vi "DecodificaAO.vi"(4 "ForzaAO_PLC":refnum<vi>, 6 "ForzaAO_Cdaq":refnum<vi>, 7 "Caratteristiche Caricate":string[][](array[string]), 8 "AO non scalati IN":T5, 9 "AO PLCs in":T4, 10 "statoAO_Cdaq in":T9, 11 "Cluster SET AO":T6) -> (0 "AO PLCs out":T4, 1 "exit":bool, 3 "statoAO_Cdaq out":T9, 5 "AO non scalati OUT":T5)   [LabVIEW 2019]
uses:
  controls/StatoAO_cdaq.ctl
  SET ARRAY AO.ctl
  SET SINGLE AO.ctl
  AO List.ctl
  TypeDef/Lista AO sistema.ctl
  controls/statoAO_plc_1.ctl
  controls/statoAO_plc_2.ctl
  controls/statoAO_plc_3.ctl
  GlobalForzaUscite.vi
  Global dati targa SINUSPENTA.vi
  Global config keb.vi
  GlobalAOInterfaccia.vi
panel:
  out "Numeric":i32
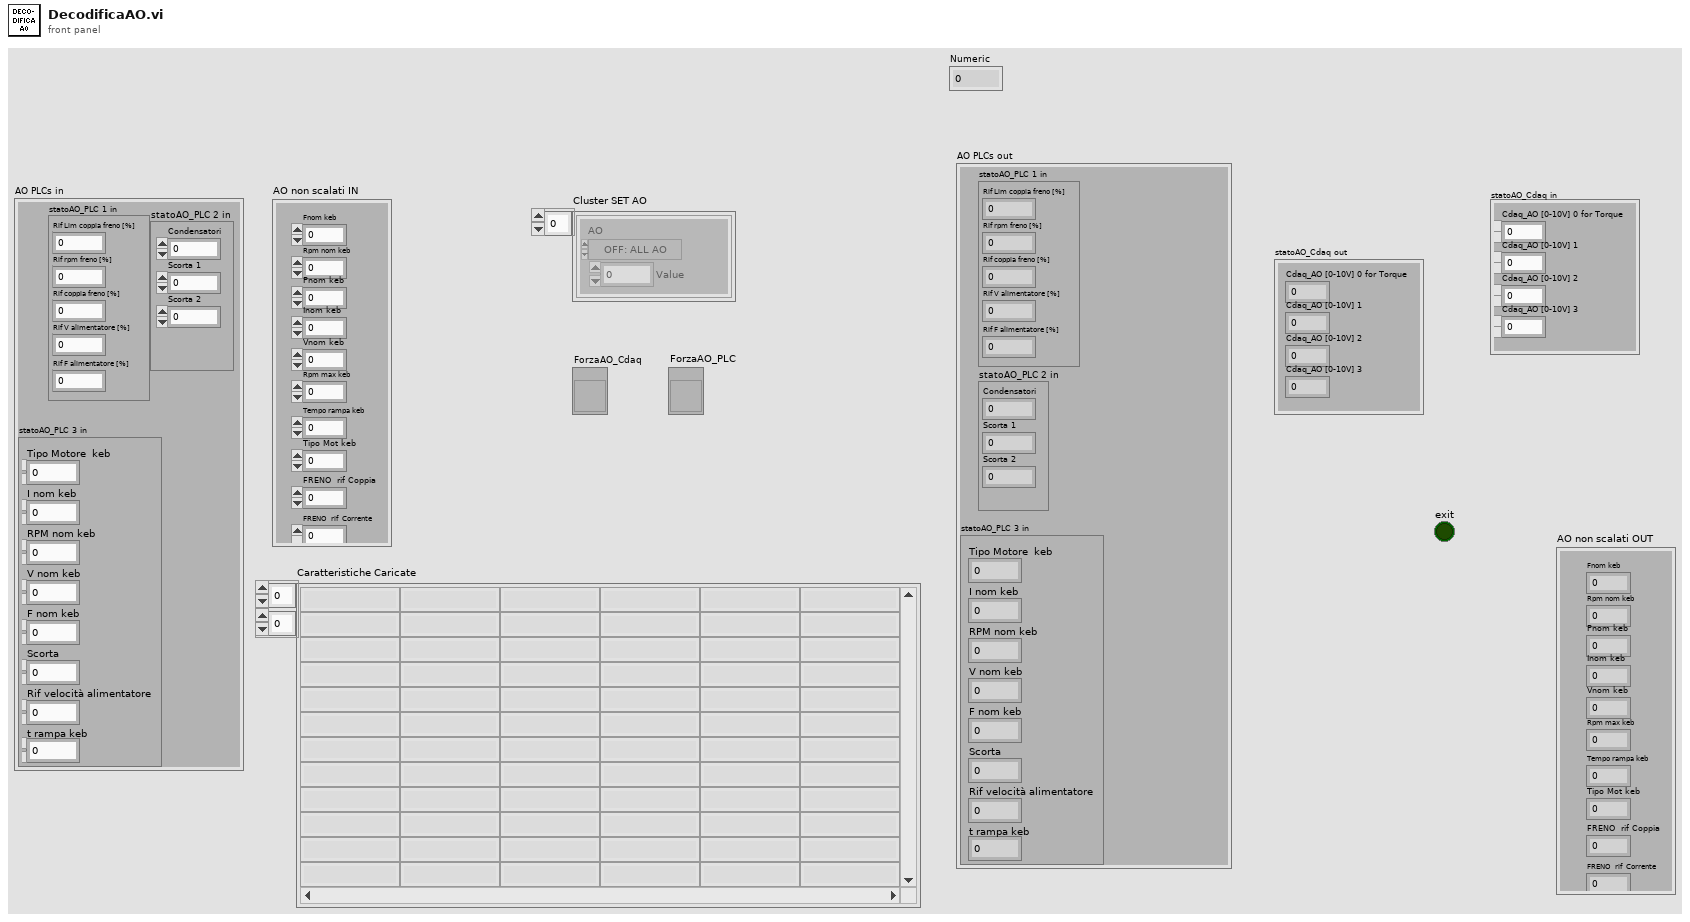
[diagram p1: front panel]
types:
  T1 = typedef "statoAO_plc_1.ctl" = cluster{"Rif Lim coppia freno [%]":dbl, "Rif rpm freno [%]":dbl, "Rif coppia freno [%]":dbl, "Rif V alimentatore [%]":dbl, "Rif F alimentatore [%]":dbl}
  T2 = typedef "statoAO_plc_2.ctl" = cluster{"Condensatori":dbl, "Scorta 1":dbl, "Scorta 2":dbl}
  T3 = typedef "statoAO_plc_3.ctl" = cluster{"Rif velocità alimentatore":dbl, "Scorta":dbl, "Tipo Motore  keb":dbl, "I nom keb":dbl, "RPM nom keb":dbl, "V nom keb":dbl, "F nom keb":dbl, "t rampa keb":dbl}
  T4 = cluster{"statoAO_PLC 1 in":T1, "statoAO_PLC 2 in":T2, "statoAO_PLC 3 in":T3}
  T5 = typedef "Lista AO sistema.ctl" = cluster{"FRENO1 rif vel":dbl, "FRENO1 rif Coppia":dbl, "FRENO2 rif vel":dbl, "FRENO2 rif Coppia":dbl, "ALIM1 rif V":dbl, "ALIM1 rif F":dbl, "ALIM2 rif V":dbl, "ALIM2 rif F":dbl, "ALIM3 rif V":dbl, "ALIM3 rif F":dbl, "Fnom keb":dbl, "Rpm nom keb":dbl, "Pnom keb":dbl, "Inom keb":dbl, "Vnom keb":dbl, "Rpm max keb":dbl, "Tempo rampa keb":dbl, "Tipo Mot keb":dbl, "FRENO  rif Coppia ":dbl, "FRENO  rif  Corrente":dbl}
  T6 = typedef "SET ARRAY AO.ctl" = T7[]
  T7 = typedef "SET SINGLE AO.ctl" = cluster{"AO":T8, "Value":dbl}
  T8 = typedef "AO List.ctl" = enum16{"OFF: ALL AO", "RIF VEL FRENO 1", "RIF VEL FRENO 2", "RIF VEL FRENO 3", "RIF COPPIA FRENO", "RIF COPPIA FRENO 1", "RIF COPPIA FRENO 2", "RIF COPPIA FRENO 3", "RIF CORRENTE FRENO 2", "RIF V ALIM 1", "RIF F ALIM 1", "RIF V ALIM 2", "RIF F ALIM 2", "RIF V ALIM 3", "RIF F ALIM 3", "RIF V ALIM 4", "RIF F ALIM 4", "FORZA AO PLC 3", "FORZA AO PLC 2", "FORZA AO PLC 1", "FORZA AO cDAQ", "Configura alimentatore keb", "Tempo rampa keb", "Condensatori", "Exit"}
  T9 = typedef "StatoAO_cdaq.ctl" = cluster{"Cdaq_AO [0-10V] 0 for Torque":dbl, "Cdaq_AO [0-10V] 1":dbl, "Cdaq_AO [0-10V] 2":dbl, "Cdaq_AO [0-10V] 3":dbl}
  T10 = typedef "ConfigurazioneKeb.ctl" = cluster{"Freq nom":dbl, "RPM nom":dbl, "Pot nom":dbl, "I nom":dbl, "V nom":dbl, "Rpm max":dbl, "Tipo Motore":dbl}
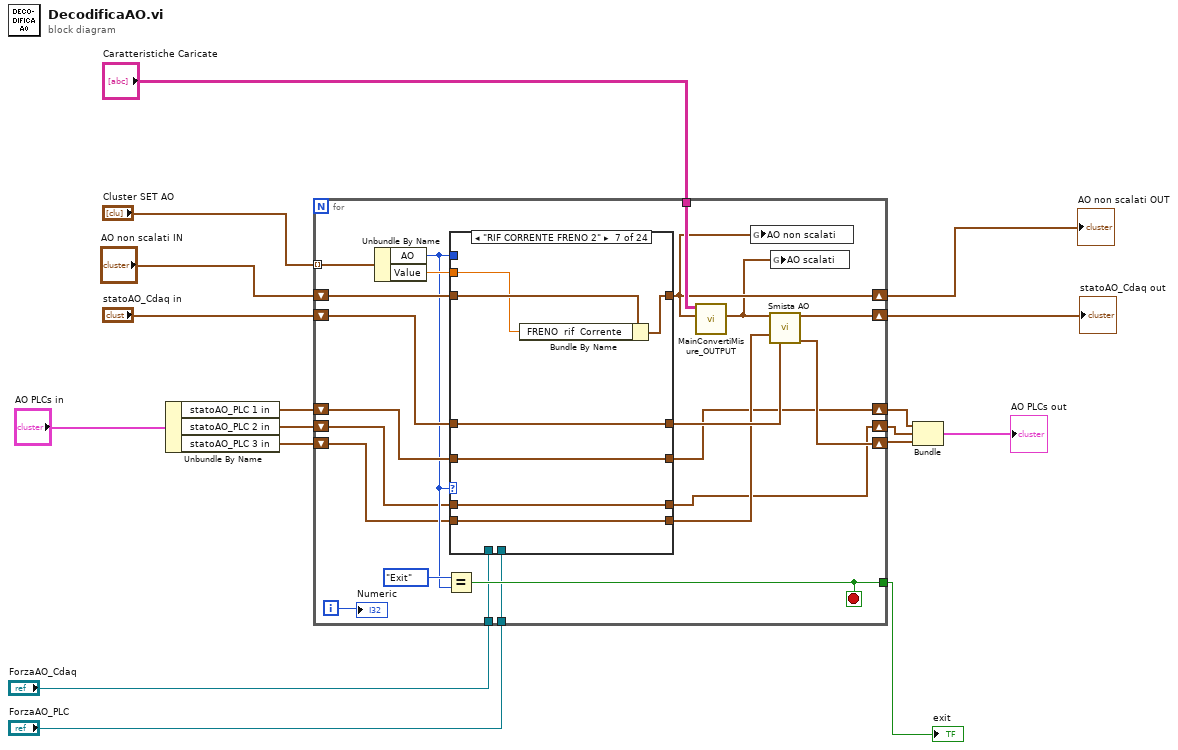
[diagram p0: block diagram]
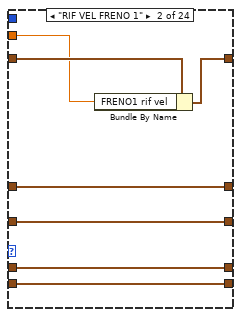
[diagram p3: hidden frame]
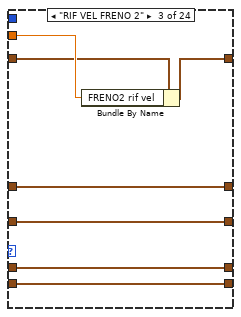
[diagram p4: hidden frame]
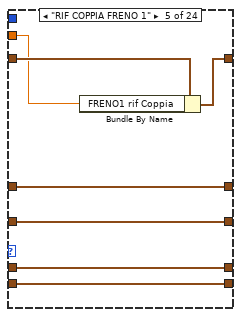
[diagram p6: hidden frame]
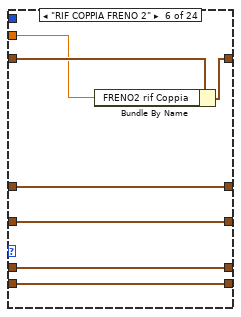
[diagram p7: hidden frame]
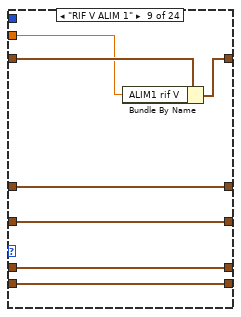
[diagram p9: hidden frame]
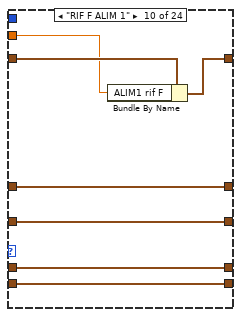
[diagram p10: hidden frame]
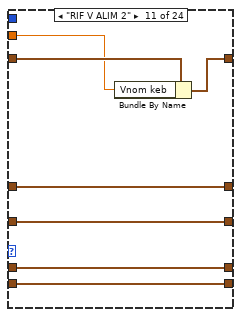
[diagram p11: hidden frame]
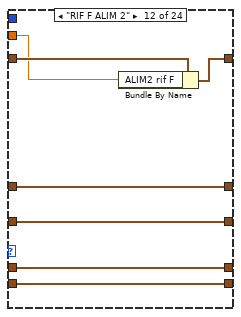
[diagram p12: hidden frame]
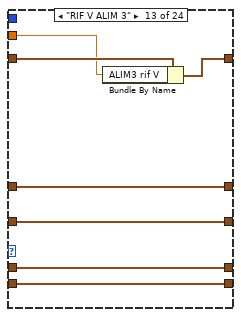
[diagram p13: hidden frame]
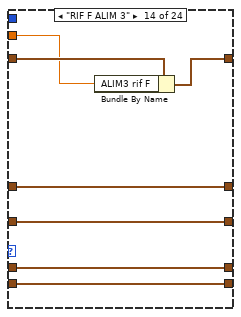
[diagram p14: hidden frame]
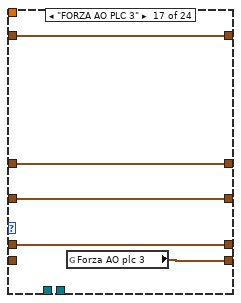
[diagram p17: hidden frame]
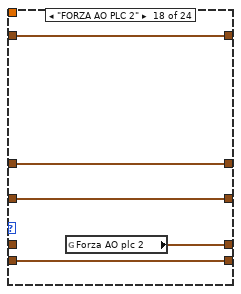
[diagram p18: hidden frame]
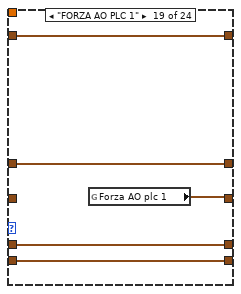
[diagram p19: hidden frame]
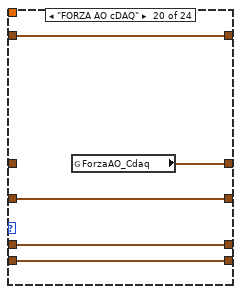
[diagram p20: hidden frame]
diagram:
  n1 = Unbundle By Name("AO PLCs in") -> ("statoAO_PLC 1 in"=w7:T1, "statoAO_PLC 2 in"=w6:T2, "statoAO_PLC 3 in"=w5:T3)
  n2 = for {
    tunnel: "Cluster SET AO" -> [w39] mode=indexing
    shift-right: [w32] -> w12
    shift-left: "statoAO_Cdaq in" -> [w31]
    shift-right: [w20] -> w4
    shift-left: w7 -> [w38]
    tunnel: [w35] -> w16
    tunnel: "ForzaAO_Cdaq" -> [w27]
    tunnel: "ForzaAO_PLC" -> [w34]
    shift-right: [w28] -> w10
    shift-left: "AO non scalati IN" -> [w33]
    tunnel: "Caratteristiche Caricate" -> [w30]
    shift-right: [w19] -> w3
    shift-left: w6 -> [w24]
    shift-right: [w25] -> w2
    shift-left: w5 -> [w23]
    i -> [w18]
    stop <- w35 stop-if-true
    n3 = Unbundle By Name(w39) -> ("AO"=w29:T8, "Value"=w37:dbl)
    n4 = Equal?(x=AO_List."Exit" ("AO"), y=w29) -> (x = y?=w35:bool)
    n5 = case shown="\"RIF CORRENTE FRENO 2\"" w29 {
      tunnel: w38 -> [w43 w51 w58 w63 w70 w77 w84 w89 w96 w103 w110 w117 w124 w131 w136 w141 w143 w151 _ w161 w176 w184 w189 w195]
      tunnel: w37 -> [_ w48 w57 _ w67 w75 w82 _ w93 w100 w107 w114 w121 w128 _ _ _ _ _ _ _ w178 w187 _]
      tunnel: w29 -> [_ _ _ _ _ _ _ _ _ _ _ _ _ _ _ _ _ _ _ _ _ _ _ _]
      tunnel: w27 -> [_ _ _ _ _ _ _ _ _ _ _ _ _ _ _ _ _ _ _ _ _ _ _ _]
      tunnel: w34 -> [_ _ _ _ _ _ _ _ _ _ _ _ _ _ _ _ _ _ _ _ _ _ _ _]
      tunnel: w33 -> [w44 w50 w56 w61 w69 w76 w83 w87 w95 w102 w109 w116 w123 w130 w134 w139 w146 w149 w155 w160 w172 w180 w190 w196]
      tunnel: [w43 w51 w58 w63 w70 w77 w84 w89 w96 w103 w110 w117 w124 w131 w136 w141 w143 w151 w152 w161 w176 w184 w188 w195] -> w20
      tunnel: [w42 w47 w54 w62 w66 w73 w80 w88 w92 w99 w106 w113 w120 w127 w135 w140 w144 w150 w156 w157 w175 w183 w191 w194] -> w26
      tunnel: w31 -> [w42 w47 w54 w62 w66 w73 w80 w88 w92 w99 w106 w113 w120 w127 w135 w140 w144 w150 w156 _ w175 w183 w191 w194]
      tunnel: [w44 w49 w55 w61 w68 w74 w81 w87 w94 w101 w108 w115 w122 w129 w134 w139 w146 w149 w155 w160 w171 w179 w190 w196] -> w28
      tunnel: w24 -> [w41 w46 w53 w60 w65 w72 w79 w86 w91 w98 w105 w112 w119 w126 w133 w138 w145 _ w154 w159 w174 w182 w186 w193]
      tunnel: [w41 w46 w53 w60 w65 w72 w79 w86 w91 w98 w105 w112 w119 w126 w133 w138 w145 w147 w154 w159 w174 w182 w186 w193] -> w19
      tunnel: w23 -> [w40 w45 w52 w59 w64 w71 w78 w85 w90 w97 w104 w111 w118 w125 w132 w137 _ w148 w153 w158 w173 w181 w185 w192]
      tunnel: [w40 w45 w52 w59 w64 w71 w78 w85 w90 w97 w104 w111 w118 w125 w132 w137 w142 w148 w153 w158 w173 w181 w185 w192] -> w22
      frame "OFF: ALL AO", Default {
      }
      frame "RIF VEL FRENO 1" {
        n6 = Bundle By Name(cluster=w50, "FRENO1 rif vel"=w48) -> (w49:T5)
      }
      frame "RIF VEL FRENO 2" {
        n7 = Bundle By Name(cluster=w56, "FRENO2 rif vel"=w57) -> (w55:T5)
      }
      frame "RIF VEL FRENO 3" {
      }
      frame "RIF COPPIA FRENO 1" {
        n8 = Bundle By Name(cluster=w69, "FRENO1 rif Coppia"=w67) -> (w68:T5)
      }
      frame "RIF COPPIA FRENO 2" {
        n9 = Bundle By Name(cluster=w76, "FRENO2 rif Coppia"=w75) -> (w74:T5)
      }
      frame "RIF CORRENTE FRENO 2" {
        n10 = Bundle By Name(cluster=w83, "FRENO  rif  Corrente"=w82) -> (w81:T5)
      }
      frame "RIF COPPIA FRENO 3" {
      }
      frame "RIF V ALIM 1" {
        n11 = Bundle By Name(cluster=w95, "ALIM1 rif V"=w93) -> (w94:T5)
      }
      frame "RIF F ALIM 1" {
        n12 = Bundle By Name(cluster=w102, "ALIM1 rif F"=w100) -> (w101:T5)
      }
      frame "RIF V ALIM 2" {
        n13 = Bundle By Name(cluster=w109, "Vnom keb"=w107) -> (w108:T5)
      }
      frame "RIF F ALIM 2" {
        n14 = Bundle By Name(cluster=w116, "ALIM2 rif F"=w114) -> (w115:T5)
      }
      frame "RIF V ALIM 3" {
        n15 = Bundle By Name(cluster=w123, "ALIM3 rif V"=w121) -> (w122:T5)
      }
      frame "RIF F ALIM 3" {
        n16 = Bundle By Name(cluster=w130, "ALIM3 rif F"=w128) -> (w129:T5)
      }
      frame "RIF V ALIM 4" {
      }
      frame "RIF F ALIM 4" {
      }
      frame "FORZA AO PLC 3" {
        n17 = global read "GlobalForzaUscite.vi" "Forza AO plc 3"() -> (w142:T3)
      }
      frame "FORZA AO PLC 2" {
        n18 = global read "GlobalForzaUscite.vi" "Forza AO plc 2"() -> (w147:T2)
      }
      frame "FORZA AO PLC 1" {
        n19 = global read "GlobalForzaUscite.vi" "Forza AO plc 1"() -> (w152:T1)
      }
      frame "FORZA AO cDAQ" {
        n20 = global read "GlobalForzaUscite.vi" "ForzaAO_Cdaq"() -> (w157:T9)
      }
      frame "Configura alimentatore keb" {
        w162 = TRUE ("Dati targa KEB Inviati")
        n21 = global read "Global config keb.vi" "Configurazione keb"() -> (w170:T10)
        n22 = Unbundle By Name(w170) -> ("Freq nom"=w169:dbl, "RPM nom"=w168:dbl, "Pot nom"=w167:dbl, "I nom"=w166:dbl, "V nom"=w165:dbl, "Rpm max"=w164:dbl, "Tipo Motore"=w163:dbl)
        n23 = global write "Global dati targa SINUSPENTA.vi" "Tentativo invio dati KEB"(w162) -> ()
        n24 = global write "Global dati targa SINUSPENTA.vi" "Dati targa KEB Inviati"(w162) -> ()
        n25 = Bundle By Name(cluster=w172, "Fnom keb"=w169, "Rpm nom keb"=w168, "Pnom keb"=w167, "Inom keb"=w166, "Vnom keb"=w165, "Rpm max keb"=w164, "Tipo Mot keb"=w163) -> (w171:T5)
      }
      frame "Tempo rampa keb" {
        n26 = Bundle By Name(cluster=w180, "Tempo rampa keb"=w178) -> (w179:T5)
        n27 = global write "Global dati targa SINUSPENTA.vi" "Tempo rampa KEB inviato"(TRUE ("Tempo rampa SINUS inviato")) -> ()
      }
      frame "Condensatori" {
        n28 = Bundle By Name(cluster=w189, "Rif Lim coppia freno [%]"=w187) -> (w188:T1)
      }
      frame "Exit" {
      }
    }
    n29 = call "MainConvertiMisure_OUTPUT.vi"("AO non scalati"=w28, "Caratteristiche Caricate"=w30) -> ("AO scalati"=w21:T5)  [unwired: 9 in]
    n30 = global write "GlobalAOInterfaccia.vi" "AO non scalati"(w28) -> ()
    n31 = call "Smista AO.vi"("AO scalati IN"=w21, "Forza AO plc_3"=w22, "Forza AO cdaq"=w26) -> ("statoAO_Cdaq out"=w32:T9, "statoAO_PLC 3 out"=w25:T3)  [unwired: 11 in]
    n32 = global write "GlobalAOInterfaccia.vi" "AO scalati"(w21) -> ()
    "Numeric" <- w18
  }
  "statoAO_Cdaq out" <- w12
  "exit" <- w16
  "AO non scalati OUT" <- w10
  n33 = Bundle("statoAO_PLC 1 in"=w4, "statoAO_PLC 2 in"=w3, "statoAO_PLC 3 in"=w2) -> (→"AO PLCs out":T4)  [unwired: 1 in]
